vi "Find Tunnel Wire.vi"(10 "Wires":T1[](array[typedef]), 11 "termUUID":string) -> (1 "other_end":string, 2 "Index":i32, 3 "destination terminal":string)   [LabVIEW 2025]
uses:
  Controls/wire.ctl
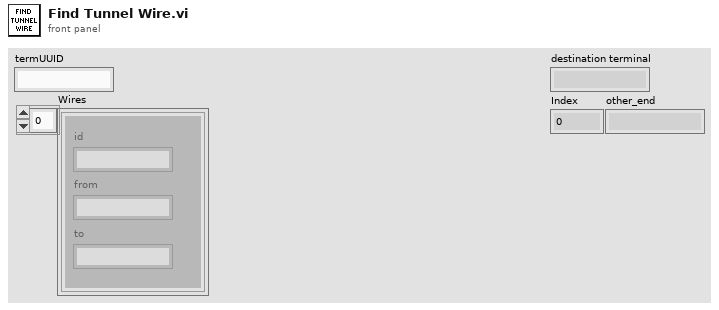
[diagram p1: front panel]
types:
  T1 = typedef "wire.ctl" = cluster{"id":string, "from":string, "to":string}
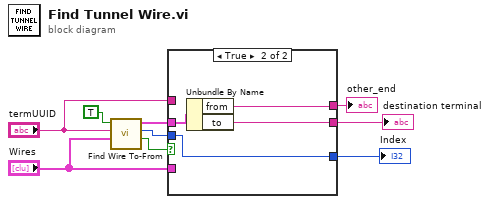
[diagram p0: block diagram]
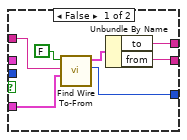
[diagram p2: hidden frame]
diagram:
  n1 = call "Find Wire To-From.vi"("Wires"="Wires", "termUUID"="termUUID", "From UUID?"=TRUE) -> ("Found"=w8:bool, "Index"=w5:i32, "Wire"=w7:T1)  [unwired: 6 in]
  n2 = case shown="True" w8 {
    tunnel: w7 -> [_ w20]
    tunnel: [w12 w19] -> w6
    tunnel: w5 -> [_ w18]
    tunnel: [w11 w18] -> w4
    tunnel: "Wires" -> [w15 _]
    tunnel: "termUUID" -> [w14 _]
    tunnel: [w10 w17] -> w1
    frame False {
      n3 = call "Find Wire To-From.vi"("Wires"=w15, "termUUID"=w14, "From UUID?"=FALSE) -> ("Index"=w11:i32, "Wire"=w13:T1)  [unwired: 6 in, 1 out]
      n4 = Unbundle By Name(w13) -> ("to"=w10:string, "from"=w12:string)
    }
    frame True {
      n5 = Unbundle By Name(w20) -> ("from"=w17:string, "to"=w19:string)
    }
  }
  "destination terminal" <- w6
  "Index" <- w4
  "other_end" <- w1
